vi "vipm_SyncVIPMPackageLibrary.vi"(8 "error in (no error)":errorcluster, 11 "CommandLine":string[](array[string])) -> (0 "error out":errorcluster, 2 "test details":string, 3 "output to action":string)   [LabVIEW 2014]
uses:
  _lvcicd/_lvcicd_support_2014.lvlib
  <vilib>/JKI/VIPM API/VIPM API_vipm_api.lvlib
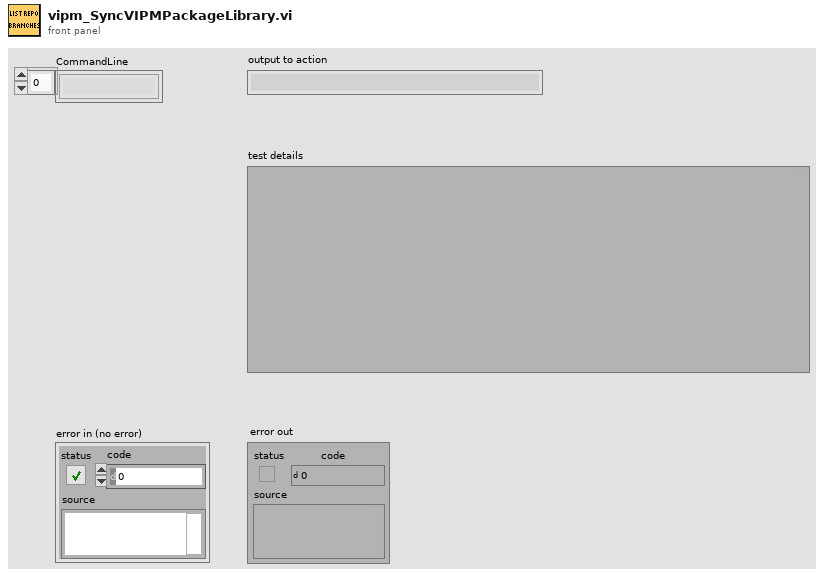
[diagram p1: front panel]
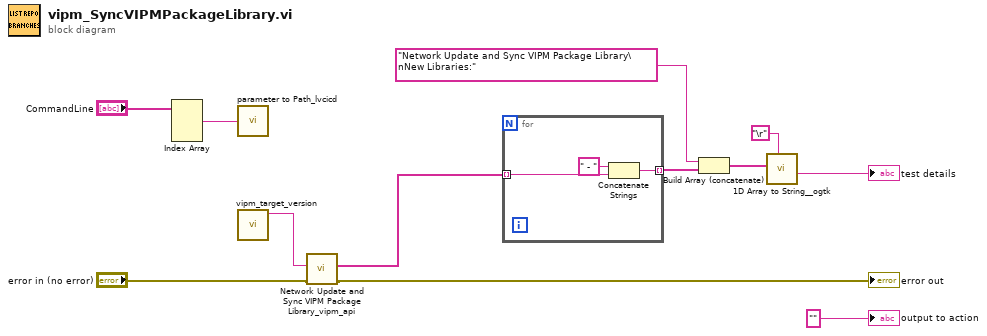
[diagram p0: block diagram]
diagram:
  n1 = Index Array(array="CommandLine") -> (element #1=w11:string)  [unwired: 3 in, 2 out]
  n2 = call "parameter to Path_lvcicd.vi"("String"=w11) -> ()  [unwired: 1 out]
  n3 = call "vipm_target_version.vi"() -> ("vipm Taget version"=w9:string)  [unwired: 11 in]
  n4 = call <vilib>:"Network Update and Sync VIPM Package Library_vipm_api.vi"("error in (no error)"="error in (no error)", "LabVIEW Version"=w9) -> ("error out"=→"error out":errorcluster, "New Package Updates"=w2:string[])  [unwired: 8 in]
  n5 = for {
    tunnel: w2 -> [w14] mode=indexing
    tunnel: [w15] -> w6 mode=indexing
    n6 = Concatenate Strings(" - " ("string"), w14) -> (w15:string)
  }
  n7 = Build Array (concatenate)("Network Update and Sync VIPM Package Library\nNew Libraries:" ("format string"), w6) -> (w4:string[])
  n8 = call <userlib>:"1D Array to String__ogtk.vi"("delimiter (Tab)"="\r", "Array of Strings"=w4) -> ("delimited string"=→"test details":string)  [unwired: 9 in]
  "output to action" <- "" ("test details")
